vi "setFont.vi"(0 "reference":refnum<class "Graphics.lvclass">, 1 "fontType":T2=enum."Application Font", 2 "font":T1, 5 "error in (no error)":errorcluster) -> (14 "reference out":refnum<class "Graphics.lvclass">, 19 "error out":errorcluster)   [LabVIEW 2014, in "Graphics.lvclass"]
doc: "Sets the font"
uses:
  <resource>/Framework/Providers/Open_GDS/UML/Graphics_class/Graphics.lvclass
  <resource>/Framework/Providers/Open_GDS/UML/Graphics_class/LvFontType.ctl
  <resource>/Framework/Providers/Open_GDS/UML/Graphics_class/FontType.ctl
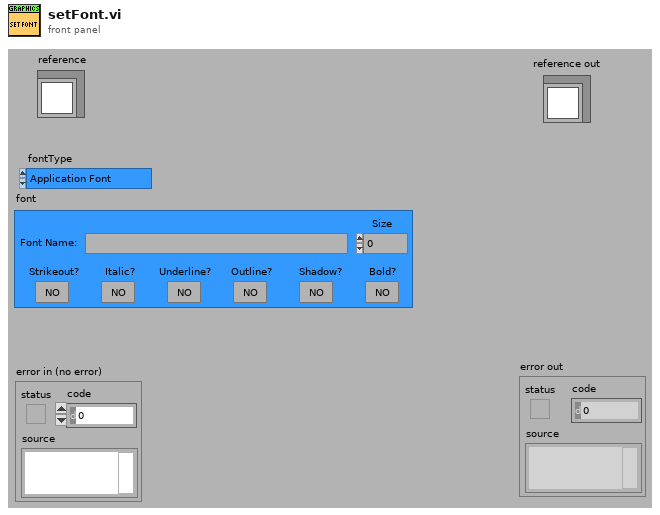
[diagram p1: front panel]
types:
  T1 = typedef "Graphics.lvclass/FontType.ctl" = cluster{"Font Name:":string, "Size":i16, "Strikeout?":bool, "Italic?":bool, "Underline?":bool, "Outline?":bool, "Shadow?":bool, "Bold?":bool}
  T2 = typedef "Graphics.lvclass/LvFontType.ctl" = enum16{"User-specified Font", "Application Font", "System Font", "Dialog Font"}
  T3 = typedef "Graphics.lvclass/ObjectAttributes.ctl" = cluster{"drawColor":u32, "backgroundColor":u32, "font":T1, "fontType":T2, "picture":picture, "stroke":T4, "scaleX":dbl, "scaleY":dbl, "screenRef":refnum<vi>, "offsetX":dbl, "offsetY":dbl}
  T4 = typedef "Graphics.lvclass/StrokeType.ctl" = enum16{"USE_DEFAULT", "SOLID", "DOTTED"}
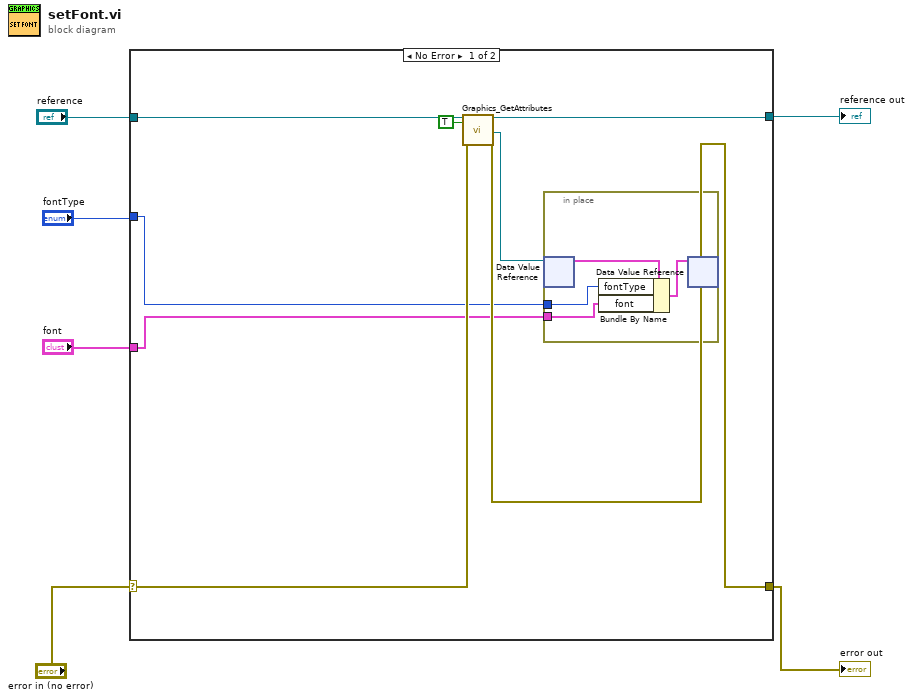
[diagram p0: block diagram]
diagram:
  n1 = case shown="No Error" "error in (no error)" {
    selector: "error in (no error)" -> [w14 w19]
    tunnel: "reference" -> [w13 w20]
    tunnel: [w12 w19] -> w4
    tunnel: [w11 w20] -> w3
    tunnel: "fontType" -> [w8 _]
    tunnel: "font" -> [w7 _]
    frame No Error {
      n2 = call <resource>:"Graphics_GetAttributes.vi"("reference in"=w13, "OnlyGetDvrReference(False)"=TRUE, "error in (no error)"=w14) -> ("reference out"=w11:refnum<class "Graphics.lvclass">, "DataRef"=w9:refnum<data-value>, "error out"=w12:errorcluster)  [unwired: 13 in, 1 out]
      n3 = in-place {
        in-place-border: w8 -> [w17]
        in-place-border: w7 -> [w16]
        n4 = in-place-dvr #1(w9) -> (w18:T3)  [unwired: 1 out]
        n5 = Bundle By Name(cluster=w18, "fontType"=w17, "font"=w16) -> (w15:T3)
        n6 = in-place-dvr #1(w15) -> ()  [unwired: 2 out]
      }
    }
    frame Error {
    }
  }
  "reference out" <- w3
  "error out" <- w4
